vi "receivePubDataCommunication.vi"(8 "error in (no error)":errorcluster, 10 "pubDataSV":T1, 11 "Cmtr in":refnum<class "Communicator.lvclass">) -> (0 "error out":errorcluster, 2 "value":variant, 3 "Cmtr out":refnum<class "Communicator.lvclass">)   [LabVIEW 2012, in "EXACommunications.lvlib" / "Communicator.lvclass"]
doc: "Reads value from PubData SV."
uses:
  Communicator.lvclass
  Typedefs/PubDataSV.ctl
  C/Program Files (x86)/National Instruments/LabVIEW 2012/user.lib/Common/ComponentModel/ComponentModel/Typedefs/CommunicationConfig.ctl
  C/Program Files (x86)/National Instruments/LabVIEW 2012/user.lib/Common/ComponentModel/ComponentModel/SVMessenger/SVMessenger.lvclass
  C/Program Files (x86)/National Instruments/LabVIEW 2012/user.lib/Common/ComponentModel/ComponentModel/Messenger/Messenger.lvclass/Messenger.ctl
  C/Program Files (x86)/National Instruments/LabVIEW 2012/user.lib/Common/ComponentModel/ComponentModel/Messenger/Messenger.lvclass
  Typedefs/EXATypedefs.lvlib
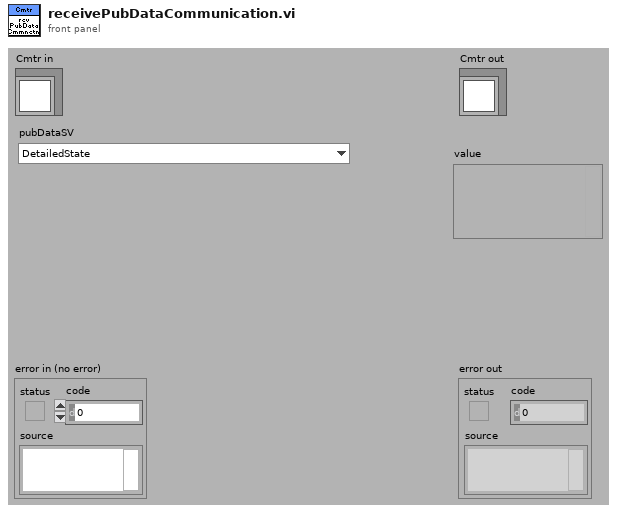
[diagram p1: front panel]
types:
  T1 = typedef "EXATypedefs.lvlib/PubDataSV.ctl" = enum16{"DetailedState", "ErrorCode", "Heartbeat", "LoopTime_ms", "LoopTimeOutOfRange", "SummaryState", "Timestamp"}
  T2 = typedef "CommunicationConfig.ctl" = cluster{"hostComputerAddress":string, "ComponentAcronym":string, "InstanceIdentifier":i32}
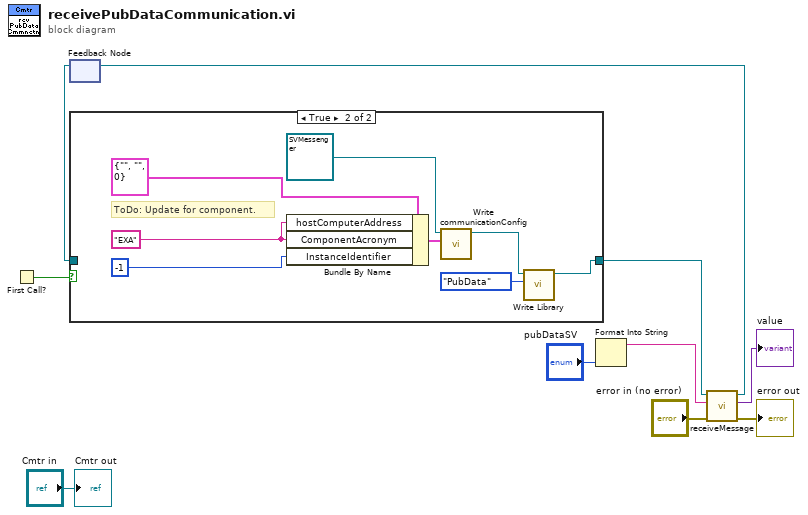
[diagram p0: block diagram]
diagram:
  n1 = First Call?() -> (First Call?: T/F=w9:bool)
  n2 = feedback #1() -> (w8:refnum<class "SVMessenger.lvclass">)  [unwired: 1 in]
  n3 = case shown="True" w9 {
    tunnel: [w11 w12] -> w6
    tunnel: w8 -> [w11 _]
    frame False {
    }
    frame True {
      w18 = "EXA" ("hostComputerAddress")
      # "ToDo: Update for component."
      n4 = Bundle By Name(cluster=T2 {"hostComputerAddress"="", "ComponentAcronym"="", "InstanceIdentifier"=0} ("sharedVariableLibrariesConfig"), "hostComputerAddress"=w18, "ComponentAcronym"=w18, "InstanceIdentifier"=-1) -> (w16:T2)
      n5 = call "Write communicationConfig.vi"("communicationConfig"=w16, "Messenger in"=refnum<class "SVMessenger.lvclass"> refnum ("SVMessenger.lvclass")) -> ("Messenger out"=w14:refnum<class "SVMessenger.lvclass">)  [unwired: 9 in]
      n6 = call "Write Library.vi"("Library"=enum16{"PubData", "SubData"}."PubData", "Messenger in"=w14) -> ("Messenger out"=w12:refnum<class "SVMessenger.lvclass">)  [unwired: 9 in]
    }
  }
  n7 = Format Into String("pubDataSV") -> (resulting string=w5:string)  [unwired: 3 in, 1 out]
  n8 = call "receiveMessage.vi"("error in (no error)"="error in (no error)", "signalName"=w5, "Messenger in"=w6) -> ("error out"=→"error out":errorcluster, "value"=→"value":variant, "Messenger out"=w1:refnum<class "SVMessenger.lvclass">)  [unwired: 5 in, 1 out]
  n9 = feedback-in #1(w1) -> ()
  "Cmtr out" <- "Cmtr in"
